vi "Sysdef.LoadFile.vi"(8 "error in (no error)":errorcluster, 11 "Path in":path) -> (0 "error out":errorcluster, 3 "SysDef":T1 {"Tree"."Properties"."Type" items=["K_STRING", "K_BOOL", "K_I32", "K_U32", "K_DOUBLE", "K_U64", "K_VARIANT", "K_DEPENDENTFILE", "K_DEPENDENTNODE", "K_DATASOURCENODE", "K_U16", "K_DBLARR", "K_U32ARR", "K_I32ARR", "K_STRINGARR", "K_DICTIONARY", "K_DICTIONARYARR"]})   [LabVIEW 2015, in "Import - Export CD Config Utility.lvlib"]
doc: "Reads the configuration file (.dat) and loads it into SysDef cluster"
uses:
  Import - Export CD Config Utility.lvlib
  _Types/SysDef.Export.ctl
  _Types/TreeItem.ctl
  _Types/TreeItem.Info.ctl
  <vilib>/NI Veristand/Custom Device API/Custom Device Channel.ctl
  <vilib>/NI Veristand/Custom Device API/Custom Device Channel Type.ctl
  <vilib>/NI Veristand/Custom Device API/Custom Device Waveform.ctl
  <vilib>/NI Veristand/Custom Device API/Custom Device Waveform DataType.ctl
  _Types/TreeItem.Property.ctl
  _Types/File.DataType.ctl
  <vilib>/NI Veristand/Custom Device API/Custom Device API.lvlib
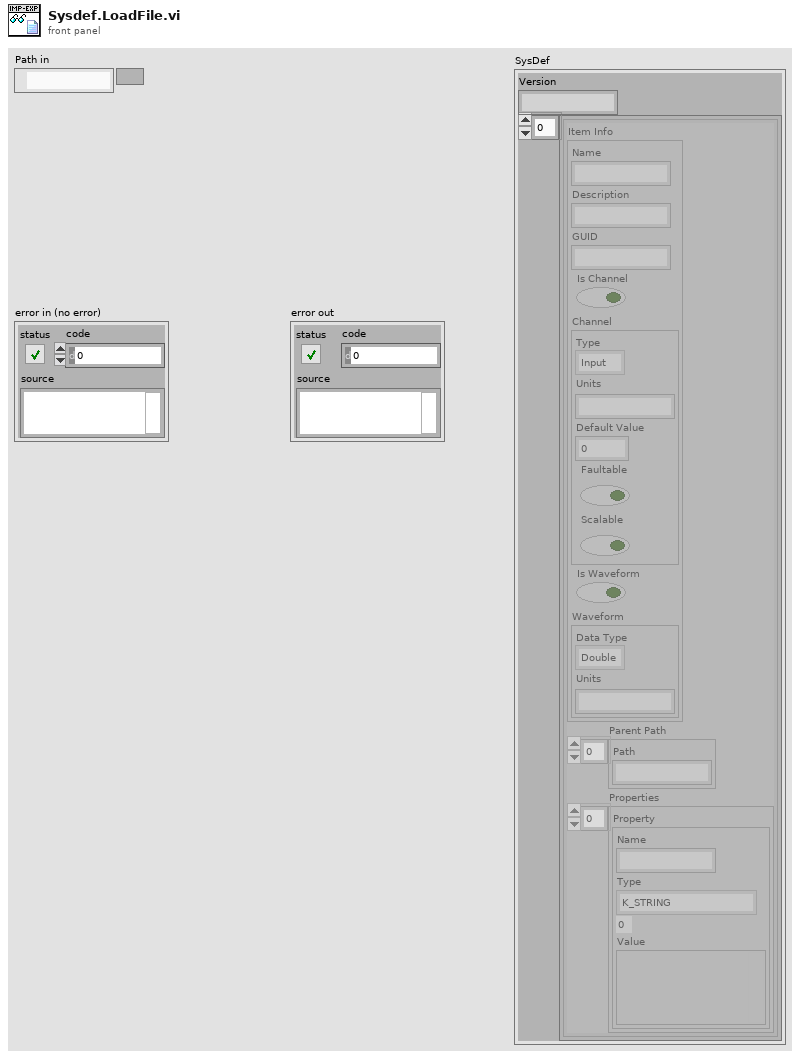
[diagram p1: front panel]
types:
  T1 = typedef "Import - Export CD Config Utility.lvlib/SysDef.Export.ctl" = cluster{"Version":string, "Tree":T2[]}
  T2 = typedef "Import - Export CD Config Utility.lvlib/TreeItem.ctl" = cluster{"Item Info":T3, "Parent Path":string[], "Properties":T8[]}
  T3 = typedef "Import - Export CD Config Utility.lvlib/TreeItem.Info.ctl" = cluster{"Name":string, "Description":string, "GUID":string, "Is Channel":bool, "Channel":T4, "Is Waveform":bool, "Waveform":T6}
  T4 = typedef "Custom Device API.lvlib/Custom Device Channel.ctl" = cluster{"Type":T5, "Units":string, "Default Value":dbl, "Faultable":bool, "Scalable":bool}
  T5 = typedef "Custom Device API.lvlib/Custom Device Channel Type.ctl" = enum16{"Input", "Output"}
  T6 = typedef "Custom Device API.lvlib/Custom Device Waveform.ctl" = cluster{"Data Type":T7, "Units":string}
  T7 = typedef "Custom Device API.lvlib/Custom Device Waveform DataType.ctl" = enum16{"Double", "Complex Double"}
  T8 = typedef "Import - Export CD Config Utility.lvlib/TreeItem.Property.ctl" = cluster{"Name":string, "Type":i32, "Value":variant}
  T9 = typedef "Import - Export CD Config Utility.lvlib/File.DataType.ctl" = cluster{"Version":string, "Data":variant}
  T10 = enum16{"open", "replace", "create", "open or create", "replace or create", "replace or create with confirmation"}
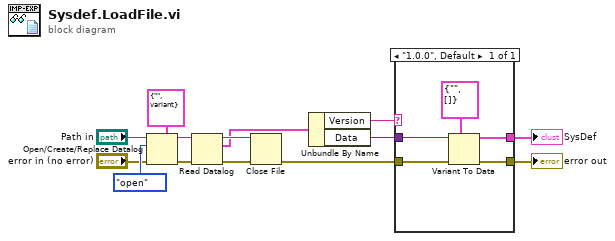
[diagram p0: block diagram]
diagram:
  n1 = Open/Create/Replace Datalog(5:T9 {"Version"="", "Data"=variant} ("Configuration"), 8:"error in (no error)", 10:T10."open" ("operation (0:open)"), 11:"Path in") -> (0:w11:errorcluster, 3:w10:refnum<k1>)  [unwired: 2 in, 1 out]
  n2 = Read Datalog(4:w11, 7:w10) -> (0:w9:errorcluster, 2:w3:T9, 3:w8:refnum<k1>)  [unwired: 1 in]
  n3 = Close File(refnum=w8, error in=w9) -> (error out=w4:errorcluster)  [unwired: 1 out]
  n4 = Unbundle By Name(w3) -> ("Version"=w2:string, "Data"=w1:variant)
  n5 = case shown="\"1.0.0\", Default" w2 {
    tunnel: [w19] -> w14
    tunnel: w4 -> [w15]
    tunnel: [w17] -> w13
    tunnel: w1 -> [w16]
    frame "1.0.0", Default {
      n6 = Variant To Data(error in=w15, type=T1 {"Version"="", "Tree"=[]} ("Export"), Variant=w16) -> (data=w17:T1, error out=w19:errorcluster)
    }
  }
  "error out" <- w14
  "SysDef" <- w13
